vi "DLPIO20 Write-Read.vi"(5 "Write Buffer":u8[](array[numeric])=[2, 40] format="%x") -> (0 "Read Buffer Out":u8[](array[numeric]) format="%x", 3 "Bytes Read":u32, 4 "Bytes Written":u32=2)   [LabVIEW 2018]
uses:
  Global 1.vi
panel:
  out "Bytes Waiting":u32
  # "Enter values in Write Buffer and run program.  \nWith a loop-back connector, the data is read back into the Read Buffer."
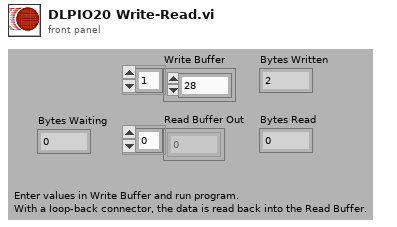
[diagram p1: front panel]
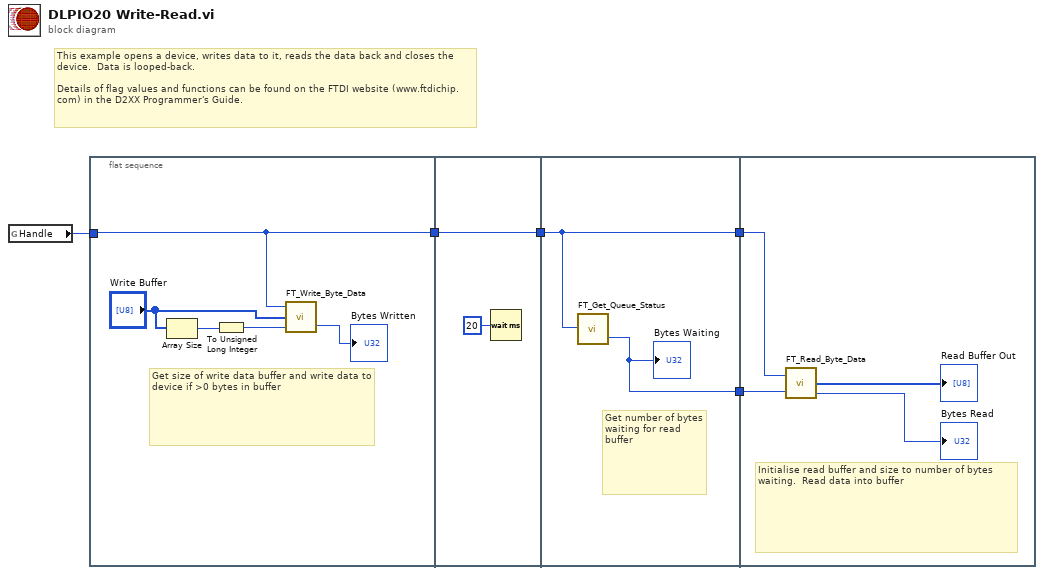
[diagram p0: block diagram]
diagram:
  # "This example opens a device, writes data to it, reads the data back and closes the device.  Data is looped-back.\n\nDetails of flag values and functions can be found on the FTDI website (www.ftdichip.com) in the D2XX Programmer's Guide."
  n1 = global read "Global 1.vi" "Handle"() -> (w1:u64)
  n2 = flat-sequence {
    tunnel: [w6] -> w2
    tunnel: w1 -> [w6]
    tunnel: w2 -> [w12]
    tunnel: [w12] -> w5
    tunnel: w5 -> [w14]
    tunnel: [w14] -> w4
    tunnel: [w13] -> w3
    tunnel: w4 -> [w17]
    tunnel: w3 -> [w15]
    frame #0 {
      # "Get size of write data buffer and write data to device if >0 bytes in buffer"
      n3 = Array Size(array="Write Buffer") -> (size(s)=w7:i32)
      n4 = To Unsigned Long Integer(number=w7) -> (unsigned 32bit integer=w8:u32)
      n5 = call "FT_Write_Byte_Data.vi"("Bytes To Write"=w8, "Buffer"="Write Buffer", "Handle"=w6) -> ("Bytes Written"=→"Bytes Written":u32)  [unwired: 1 out]
    }
    frame #1 {
      n6 = Wait (ms)(milliseconds to wait=u32 20) -> ()  [unwired: 1 out]
    }
    frame #2 {
      # "Get number of bytes waiting for read buffer"
      n7 = call "FT_Get_Queue_Status.vi"("Handle"=w14) -> ("Bytes Waiting"=w13:u32)  [unwired: 1 out]
      "Bytes Waiting" <- w13
    }
    frame #3 {
      # "Initialise read buffer and size to number of bytes waiting.  Read data into buffer"
      n8 = call "FT_Read_Byte_Data.vi"("Handle"=w17, "Bytes To Read"=w15) -> ("Read Data"=→"Read Buffer Out":u8[], "Bytes Read"=→"Bytes Read":u32)  [unwired: 1 out]
    }
  }
